vi "Read Source file name.vi"(11 "ProjectItem in":refnum<class "ProjectItem.lvclass">) -> (2 "Source file name":string, 3 "ProjectItem out":refnum<class "ProjectItem.lvclass">)   [LabVIEW 2019, in "SolutionBuilder.lvlib" / "ProjectItem.lvclass"]
uses:
  ProjectItem.lvclass
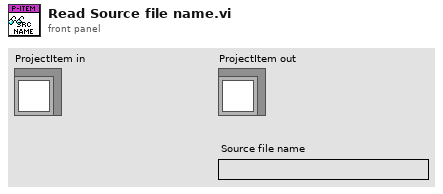
[diagram p1: front panel]
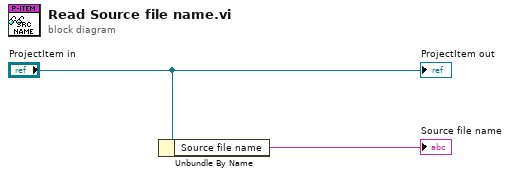
[diagram p0: block diagram]
diagram:
  n1 = Unbundle By Name("ProjectItem in") -> ("Source file name"=→"Source file name":string)
  "ProjectItem out" <- "ProjectItem in"
